vi "Run_apple_script.vi"(1 "file names":string[](array[string])) -> (0 "error string":string)   [LabVIEW 2010]
panel:
  in  "type specifier VI Refnum (for type only)":refnum<vi>
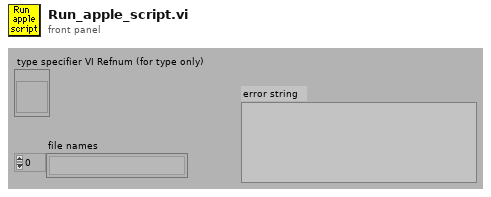
[diagram p1: front panel]
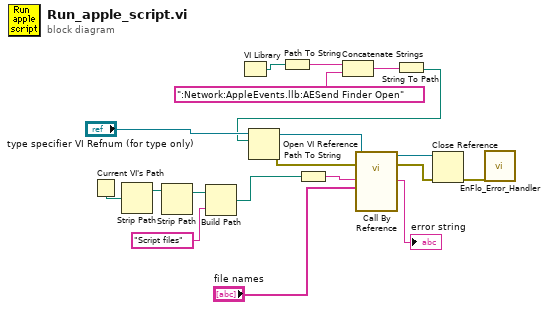
[diagram p0: block diagram]
diagram:
  n1 = Current VI's Path() -> (path=w6:path)
  n2 = Strip Path(path=w6) -> (stripped path=w16:path)  [unwired: 1 out]
  n3 = Strip Path(path=w16) -> (stripped path=w17:path)  [unwired: 1 out]
  n4 = Build Path(base path=w17, name or relative path="Script files") -> (appended path=w19:path)
  n5 = VI Library() -> (path=w4:path)
  n6 = Path To String(path=w4) -> (string=w3:string)
  n7 = Path To String(path=w19) -> (string=w15:string)
  n8 = Concatenate Strings(w3, ":Network:AppleEvents.llb:AESend Finder Open") -> (w1:string)
  n9 = String To Path(string=w1) -> (path=w5:path)
  n10 = Open VI Reference(type specifier VI Refnum (for type only)="type specifier VI Refnum (for type only)", vi path=w5) -> (vi reference=w7:refnum<vi>, error out=w8:errorcluster)  [unwired: 4 in]
  n11 = call-by-ref "?"(reference=w7, error in=w8, "file names"="file names", "Full path of folder containing files"=w15) -> (reference out=w12:refnum<vi>, error out=w13:errorcluster, "error string"=→"error string":string)  [unwired: 4 in, 1 out]
  n12 = Close Reference(reference=w12, error in (no error)=w13) -> (error out=w14:errorcluster)
  n13 = call "EnFlo_Error_Handler.vi"("error in (no error)"=w14) -> ()  [unwired: 2 in, 3 out]
